vi "GetPlugin.vi"(8 "error in (no error)":errorcluster, 10 "name or relative path":string, 11 "Serializer.lvlib:Serial.lvclass":refnum<class "Serial.lvclass">) -> (0 "error out":errorcluster, 3 "serialClass":refnum<class "Serial.lvclass">)   [LabVIEW 2015, in "Serializer.lvlib"]
uses:
  Serializer.lvlib
  OOP/Serial/Base/Serial.lvclass
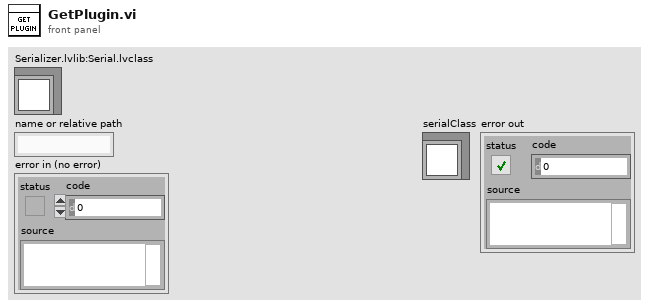
[diagram p1: front panel]
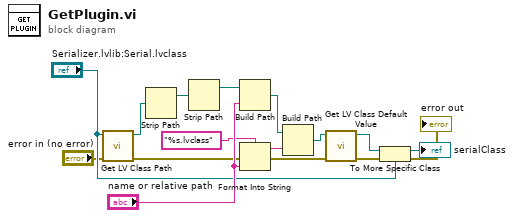
[diagram p0: block diagram]
diagram:
  n1 = call <vilib>:"Get LV Class Path.vi"("error in (no error)"="error in (no error)", "object"="Serializer.lvlib:Serial.lvclass") -> ("error out"=w5:errorcluster, "class path"=w16:path)  [unwired: 8 in]
  n2 = Strip Path(path=w16) -> (stripped path=w14:path)  [unwired: 1 out]
  n3 = Strip Path(path=w14) -> (stripped path=w13:path)  [unwired: 1 out]
  n4 = Build Path(base path=w13, name or relative path="name or relative path") -> (appended path=w11:path)
  n5 = Format Into String(format string="%s.lvclass", error in=w5, "name or relative path") -> (resulting string=w8:string, error out=w4:errorcluster)  [unwired: 1 in]
  n6 = Build Path(base path=w11, name or relative path=w8) -> (appended path=w12:path)
  n7 = call <vilib>:"Get LV Class Default Value.vi"("error in (no error)"=w4, "class path"=w12) -> ("error out"=w15:errorcluster, "object"=w7:refnum<class>)  [unwired: 8 in]
  n8 = To More Specific Class(target class="Serializer.lvlib:Serial.lvclass", reference=w7, error in=w15) -> (specific class reference=→"serialClass":refnum<class "Serial.lvclass">, error out=→"error out":errorcluster)
